vi "66xxA Set OVP OCP.vi"(6 "channel (1)":u8=1 min=1 max=4 step=1, 8 "error in (no error)":errorcluster, 9 "overcurrent\nprotection (F:off)":bool, 10 "overvoltage\nprotection (23.0 V)":dbl=23.0 format="%.1f", 11 "VISA resource name":refnum<visa-resource-name>) -> (0 "error out":errorcluster, 3 "VISA resource name out":refnum<visa-resource-name>)   [LabVIEW 2020, in "Agilent 6XXX Series.lvlib"]
doc: "This function sets the overvoltage protection and overcurrent protection of the HP662XA series and the HP663XA series."
uses:
  <instrlib>/Agilent 6XXX Series/Agilent 6XXX Series.lvlib
panel:
  # "HP662XA and HP663XA series only"
  # "on\noff"
  # "*662xA only"
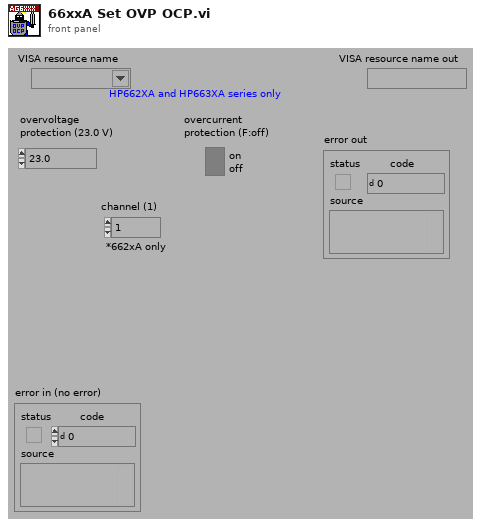
[diagram p1: front panel]
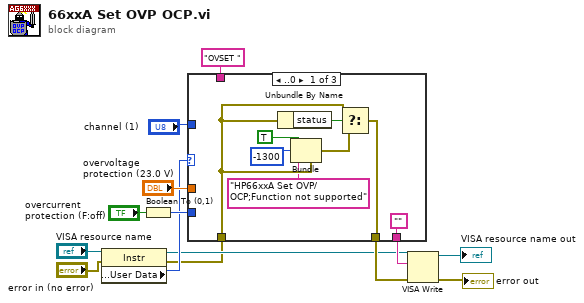
[diagram p0: block diagram]
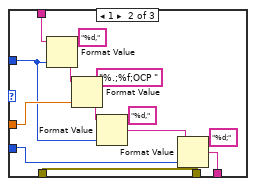
[diagram p2: hidden frame]
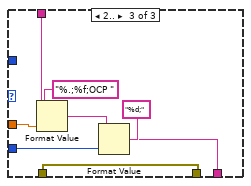
[diagram p3: hidden frame]
diagram:
  n1 = property class="Instr"(reference="VISA resource name", error in="error in (no error)") -> (reference out=w2:refnum<visa-resource-name>, error out=w1:errorcluster, "General Settings:User Data"=w3:u32)
  n2 = Boolean To (0,1)(Boolean="overcurrent\nprotection (F:off)") -> (0, 1=w6:i16)
  n3 = case shown="..0" w3 {
    tunnel: "OVSET " -> [_ w32 w42]
    tunnel: ["" w34 w37] -> w14
    tunnel: "overvoltage\nprotection (23.0 V)" -> [_ w26 w39]
    tunnel: w6 -> [_ w23 w38]
    tunnel: "channel (1)" -> [_ w25 _]
    tunnel: w1 -> [w19 w24 w36]
    tunnel: [w17 w24 w36] -> w7
    frame ..0 {
      n4 = Unbundle By Name(w19) -> ("status"=w22:bool)
      n5 = Bundle(cluster=w19, "status"=TRUE, "code"=-1300, "source"="HP66xxA Set OVP/OCP;Function not supported") -> (w18:errorcluster)
      n6 = Select(t=w19, s=w22, f=w18) -> (s? t:f=w17:errorcluster)
    }
    frame 1 {
      n7 = Format Value(string ("")=w32, format string="%d,", value (0)=w25) -> (output string=w30:string)
      n8 = Format Value(string ("")=w30, format string="%.;%f;OCP ", value (0)=w26) -> (output string=w27:string)
      n9 = Format Value(string ("")=w27, format string="%d,", value (0)=w25) -> (output string=w28:string)
      n10 = Format Value(string ("")=w28, format string="%d;", value (0)=w23) -> (output string=w34:string)
    }
    frame 2.. {
      n11 = Format Value(string ("")=w42, format string="%.;%f;OCP ", value (0)=w39) -> (output string=w41:string)
      n12 = Format Value(string ("")=w41, format string="%d;", value (0)=w38) -> (output string=w37:string)
    }
  }
  n13 = VISA Write(VISA resource name=w2, write buffer=w14, error in (no error)=w7) -> (VISA resource name out=→"VISA resource name out":refnum<visa-resource-name>, error out=→"error out":errorcluster)  [unwired: 1 out]
